vi "SSL_Read.vi"(8 "error in (no error)":errorcluster, 10 "SSL_Connection":T1, 11 "bytes to read":i32) -> (0 "error out":errorcluster, 2 "SSL_Connection 2":T1, 3 "data out":u8[](array[numeric]) format="%x")   [LabVIEW 2015, in "AWS_IoT.lvlib"]
uses:
  AWS_IoT.lvlib
  Controls/SSL_Connection.ctl
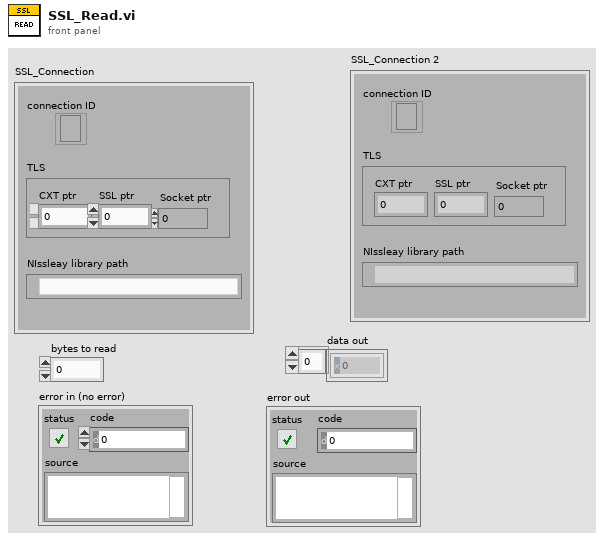
[diagram p1: front panel]
types:
  T1 = typedef "AWS_IoT.lvlib/SSL_Connection.ctl" = cluster{"connection ID":refnum<k5>, "TLS":cluster{"CXT ptr":i32, "SSL ptr":i32, "Socket ptr":u64}, "NIssleay library path":path}
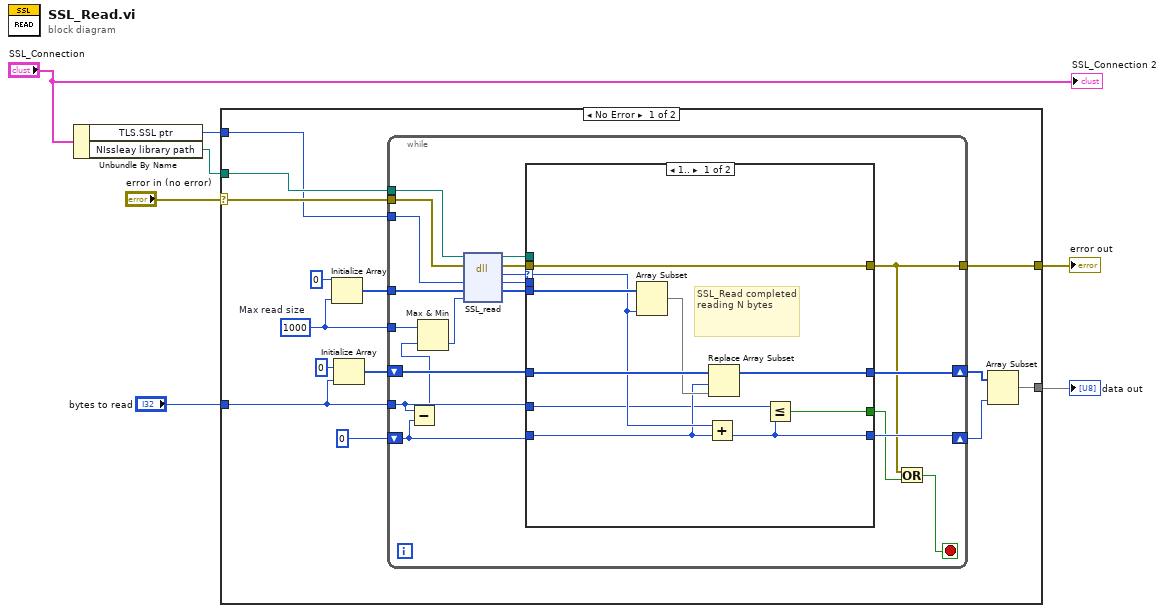
[diagram p0: block diagram]
diagram:
  n1 = Unbundle By Name("SSL_Connection") -> ("TLS.SSL ptr"=w4:i32, "NIssleay library path"=w6:path)
  n2 = case shown="No Error" "error in (no error)" {
    selector: "error in (no error)" -> [w20 w55]
    tunnel: w6 -> [w21 _]
    tunnel: w4 -> [w19 _]
    tunnel: "bytes to read" -> [w14 _]
    tunnel: [w9 _] -> w2
    tunnel: [w8 w55] -> w1
    frame No Error {
      w16 = 1000  # Max read size
      n3 = Initialize Array(u8 0 ("element"), w16) -> (w17:u8[])
      n4 = Initialize Array(u8 0 ("element"), w14) -> (w13:u8[])
      n5 = while {
        tunnel: w21 -> [w41]
        tunnel: w20 -> [w40]
        tunnel: w19 -> [w39]
        tunnel: w14 -> [w30]
        tunnel: w17 -> [w34]
        tunnel: w16 -> [w33]
        shift-right: [w31] -> w11
        shift-left: w13 -> [w32]
        shift-right: [w25] -> w10
        shift-left: 0 -> [w26]
        tunnel: [w23] -> w8
        stop <- w24 stop-if-true
        n6 = Subtract(x=w30, y=w26) -> (x-y=w29:i32)
        n7 = Max & Min(x=w33, y=w29) -> (min(x,y)=w35:i32)  [unwired: 1 out]
        n8 = dll-call lib="NIssleay32.*" fn="SSL_read"(path in=w41, error in=w40, "SSL"=w39, "stringBuf"=w34, "stringLen"=w35) -> (path out=w36:path, error out=w37:errorcluster, "noOfBytes"=w38:i32, "SSL"=w27:i32, "stringBuf"=w28:u8[])  [unwired: 2 in]
        n9 = case shown="1.." w38 {
          selector: w38 -> [w46 _]
          tunnel: w36 -> [_ _]
          tunnel: w37 -> [w51 w54]
          tunnel: [w51 w54] -> w23
          tunnel: [w42 _] -> w22
          tunnel: w28 -> [w50 _]
          tunnel: w32 -> [w49 w53]
          tunnel: [w48 w53] -> w31
          tunnel: w26 -> [w45 w52]
          tunnel: [w44 w52] -> w25
          tunnel: w30 -> [w43 _]
          tunnel: w27 -> [_ _]
          frame 1.. {
            # "SSL_Read completed reading N bytes"
            n10 = Array Subset(array=w50, length=w46) -> (w47:u8[])  [unwired: 1 in]
            n11 = Add(x=w46, y=w45) -> (x+y=w44:i32)
            n12 = Replace Array Subset(array=w49, new element=w47, index=w45) -> (w48:u8[])
            n13 = Less Or Equal?(x=w43, y=w44) -> (x <= y?=w42:bool)
          }
          frame 0, Default {
          }
        }
        n14 = Or(x=w23, y=w22) -> (x .or. y?=w24:bool)
      }
      n15 = Array Subset(array=w11, length=w10) -> (w9:u8[])  [unwired: 1 in]
    }
    frame Error {
    }
  }
  "data out" <- w2
  "error out" <- w1
  "SSL_Connection 2" <- "SSL_Connection"
